vi "TF_Complex_toMagPhase.vi"(11 "TF Corr Rx FFT Mag":T1) -> (0 "phase":dbl[](array[numeric]), 1 "magnitude":dbl[](array[numeric]), 2 "TF Phase":cluster{"f0":dbl, "df":dbl, "magnitude":dbl[]}, 3 "TF Mag":cluster{"f0":dbl, "df":dbl, "magnitude":dbl[]}, 4 "Freq array":dbl[](array[numeric]), 5 "PSD":dbl[](array[numeric]), 6 "TF PSD":cluster{"f0":dbl, "df":dbl, "magnitude":dbl[]})   [LabVIEW 2021]
panel:
  out "Waveform Graph":cluster{"f0":dbl, "df":dbl, "magnitude":dbl[]}(graph)
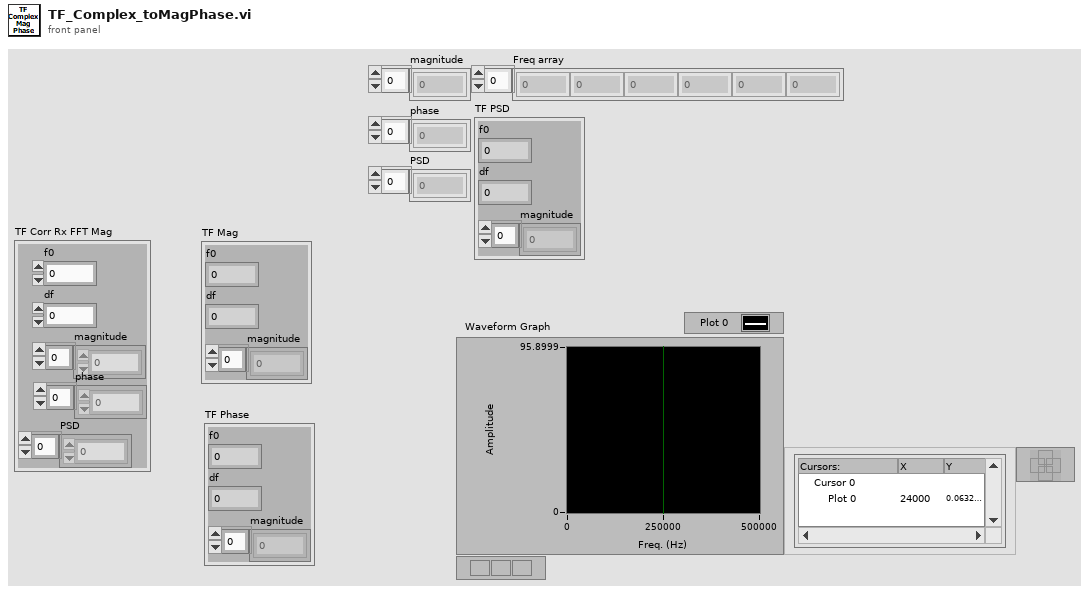
[diagram p1: front panel]
types:
  T1 = cluster{"f0":dbl, "df":dbl, "magnitude":dbl[], "phase":dbl[], "PSD":dbl[]}
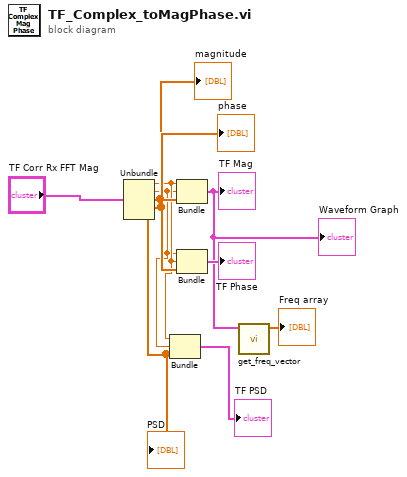
[diagram p0: block diagram]
diagram:
  n1 = Unbundle("TF Corr Rx FFT Mag") -> ("f0"=w5:dbl, "df"=w4:dbl, "magnitude"=w7:dbl[], "phase"=w9:dbl[], "PSD"=w3:dbl[])
  "magnitude" <- w7
  "phase" <- w9
  "PSD" <- w3
  n2 = Bundle("f0"=w5, "df"=w4, "PSD"=w3) -> (→"TF PSD":cluster{"f0":dbl, "df":dbl, "PSD":dbl[]})  [unwired: 1 in]
  n3 = Bundle("f0"=w5, "df"=w4, "magnitude"=w7) -> (w1:cluster{"f0":dbl, "df":dbl, "magnitude":dbl[]})  [unwired: 1 in]
  "TF Mag" <- w1
  "Waveform Graph" <- w1
  n4 = Bundle("df"=w4, "f0"=w5, "phase"=w9) -> (→"TF Phase":cluster{"df":dbl, "f0":dbl, "phase":dbl[]})  [unwired: 1 in]
  n5 = call "get_freq_vector.vi"("FFT magnitude"=w1) -> ("Freq array"=→"Freq array":dbl[])  [unwired: 10 in]
